vi "Example Callback - PositionReached Callback.vi"(4 "PositionReached":refnum<user-event>, 5 "Event Data":T1, 6 "Control Ref":refnum<k24>, 7 "Event Common Data":T2) -> ()   [LabVIEW 2010]
uses:
  C:/tf/play/labview/Tinkerforge.dll
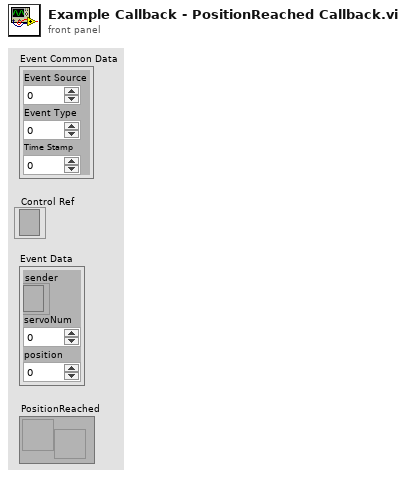
[diagram p1: front panel]
types:
  T1 = cluster{"sender":refnum<k24>, "servoNum":u8, "position":i16}
  T2 = cluster{"Event Source":i32, "Event Type":u32, "Time Stamp":u32}
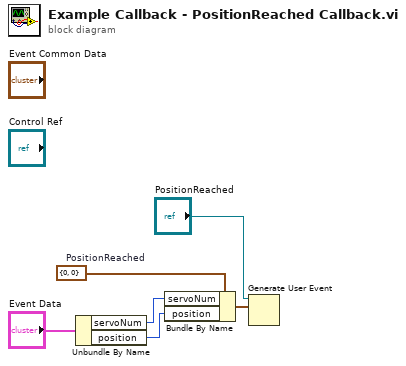
[diagram p0: block diagram]
diagram:
  w5 = cluster{"servoNum":u8, "position":i16} {"servoNum"=0, "position"=0}  # PositionReached
  n1 = Unbundle By Name("Event Data") -> ("servoNum"=w4:u8, "position"=w3:i16)
  n2 = Bundle By Name(cluster=w5, "servoNum"=w4, "position"=w3) -> (w1:cluster{"servoNum":u8, "position":i16})
  n3 = Generate User Event(user event="PositionReached", event data cluster=w1) -> ()  [unwired: 1 in, 2 out]
